vi "Page_Info_Initialize.vi"(8 "error in (no error)":errorcluster, 9 "ctlReferences":T1, 11 "AB_DepPackedLibrary in":refnum<class "AB_DepPackedLibrary.lvclass">) -> (0 "error out":errorcluster, 3 "AB_DepPackedLibrary out":refnum<class "AB_DepPackedLibrary.lvclass">)   [LabVIEW 2020, in "AB_DepPackedLibrary.lvclass"]
uses:
  <vilib>/AppBuilder/AB_Classes/DepPackedLib/AB_DepPackedLibrary.lvclass
  e:/builds/penguin/labview/branches/2020/dev/dist/vi.lib/AppBuilder/AB_Classes/Build/AB_Build.lvclass
  <resource>/Framework/Providers/Builds/AppBuilder/AB_UI_Page_Info_References.ctl
  <vilib>/AppBuilder/AB_Classes/Deployment/AB_Deployment.lvlib
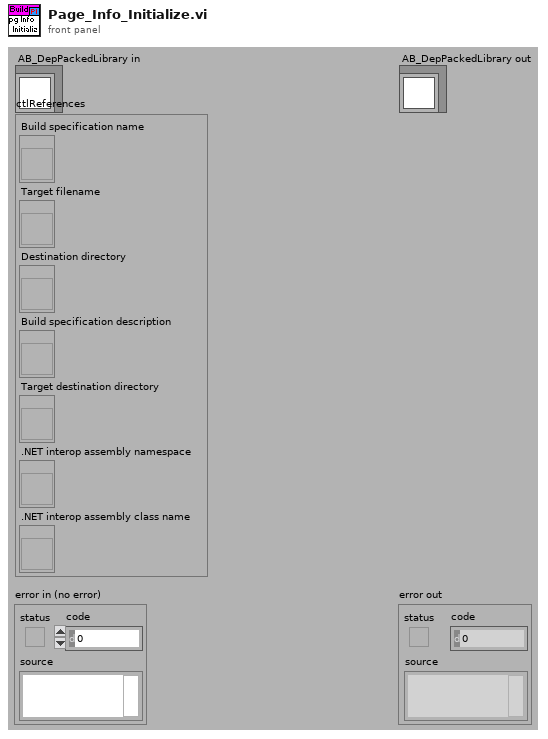
[diagram p1: front panel]
types:
  T1 = typedef "AB_UI_Page_Info_References.ctl" = cluster{"Build specification name":refnum<vi>, "Target filename":refnum<vi>, "Destination directory":refnum<vi>, "Build specification description":refnum<vi>, "Target destination directory":refnum<vi>, ".NET interop assembly namespace":refnum<vi>, ".NET interop assembly class name":refnum<vi>}
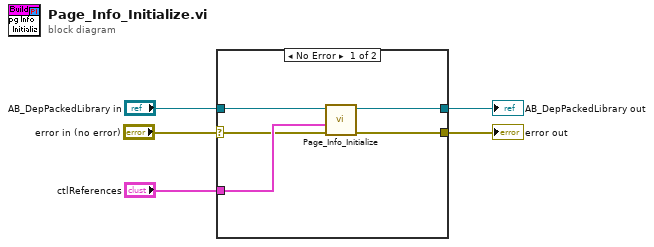
[diagram p0: block diagram]
diagram:
  n1 = case shown="No Error" "error in (no error)" {
    selector: "error in (no error)" -> [w9 w12]
    tunnel: [w8 w12] -> w4
    tunnel: [w7 w11] -> w1
    tunnel: "AB_DepPackedLibrary in" -> [w6 w11]
    tunnel: "ctlReferences" -> [w10 _]
    frame No Error {
      n2 = call <vilib>:"Page_Info_Initialize.vi"("error in (no error)"=w9, "ctlReferences"=w10, "Build in"=w6) -> ("error out"=w8:errorcluster, "Build out"=w7:refnum<class "AB_DepPackedLibrary.lvclass">)  [unwired: 7 in]
    }
    frame Error {
    }
  }
  "error out" <- w4
  "AB_DepPackedLibrary out" <- w1
